vi "StringToBool(SubVI).vi"(2 "string":string) -> (5 "Det 1":bool, 6 "Det 2":bool, 7 "Det 3":bool, 8 "Det 6":bool, 9 "Det 4":bool, 10 "Det 5":bool)   [LabVIEW 2017]
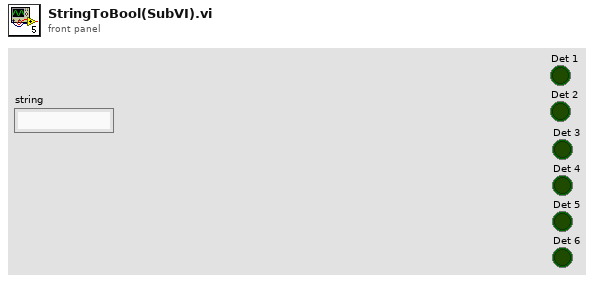
[diagram p1: front panel]
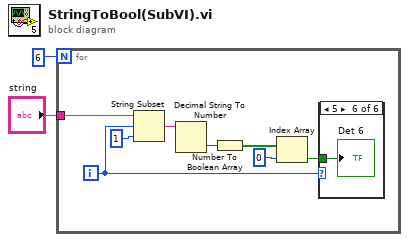
[diagram p0: block diagram]
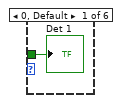
[diagram p2: hidden frame]
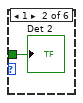
[diagram p3: hidden frame]
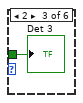
[diagram p4: hidden frame]
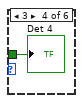
[diagram p5: hidden frame]
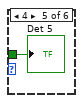
[diagram p6: hidden frame]
diagram:
  n1 = for {
    N: 6 -> [_]
    tunnel: "string" -> [w3]
    i -> [w5]
    n2 = String Subset(string=w3, offset (0)=w5, length (rest)=1 ("length (rest)")) -> (substring=w10:string)
    n3 = Decimal String To Number(string=w10) -> (number=w8:i32)  [unwired: 2 in, 1 out]
    n4 = Number To Boolean Array(number=w8) -> (Boolean array=w9:bool[])
    n5 = Index Array(array=w9, index=0) -> (element=w4:bool)
    n6 = case shown="5" w5 {
      tunnel: w4 -> [w11 w12 w13 w14 w15 w16]
      frame 0, Default {
        "Det 1" <- w11
      }
      frame 1 {
        "Det 2" <- w12
      }
      frame 2 {
        "Det 3" <- w13
      }
      frame 3 {
        "Det 4" <- w14
      }
      frame 4 {
        "Det 5" <- w15
      }
      frame 5 {
        "Det 6" <- w16
      }
    }
  }
